vi "mfd_global.vi"() -> ()   [LabVIEW 2023]
panel:
  in  "MFD_GpsControl":T1
  out "MFD_Gps":picture
  in  "MFD_BatteryControl":T2
  in  "MFD_PowerControl":T3
  in  "MFD_RcControl":T4
  out "MFD_RadioBattery":picture
  in  "MFD_Stop":bool
  out "MFD_StatusText":picture
  in  "MFD_StatusTextControl":T5(array[cluster])
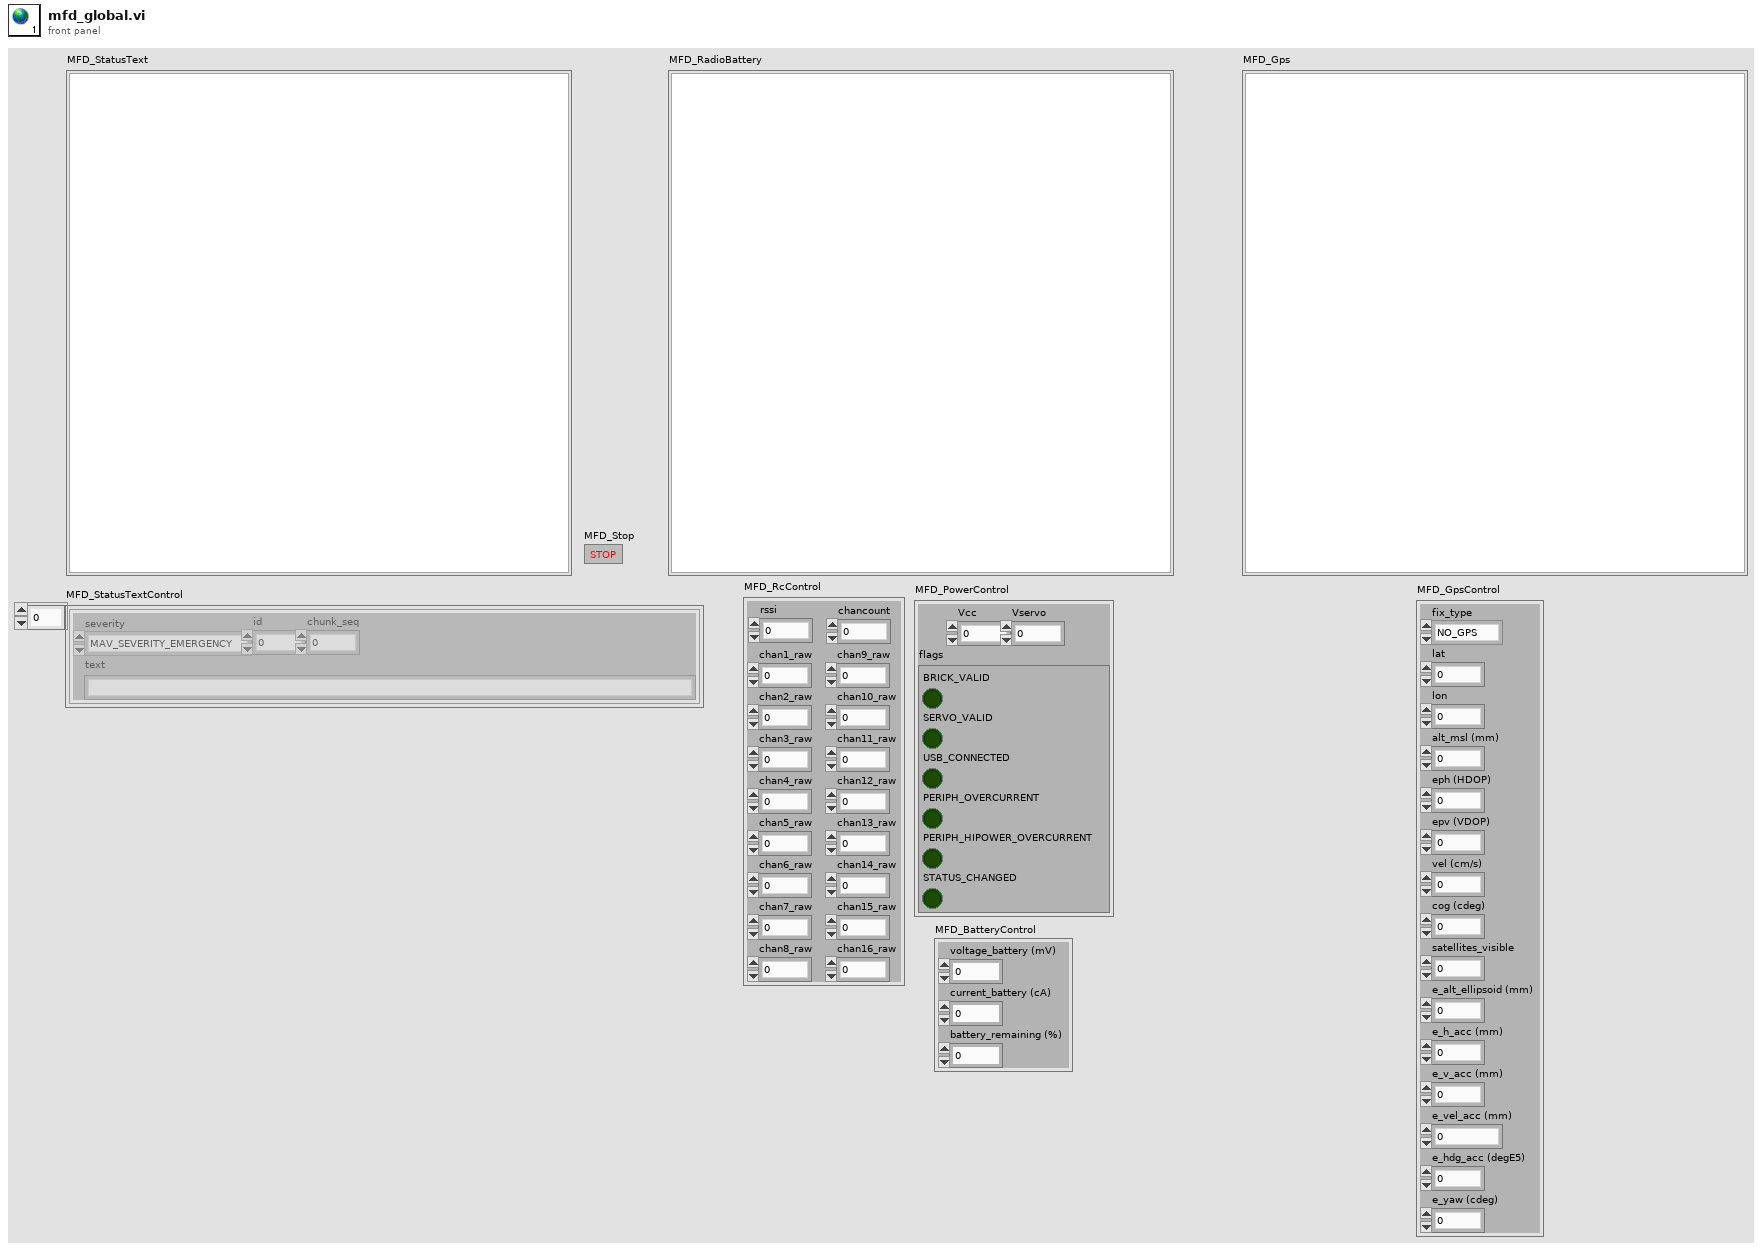
[diagram p1: front panel]
types:
  T1 = cluster{"lat":i32, "lon":i32, "alt_msl (mm)":i32, "eph (HDOP)":u16, "epv (VDOP)":u16, "vel (cm/s)":u16, "cog (cdeg)":u16, "satellites_visible":u8, "e_alt_ellipsoid (mm)":i32, "e_h_acc (mm)":u32, "e_v_acc (mm)":u32, "e_vel_acc (mm)":u32, "e_hdg_acc (degE5)":u32, "e_yaw (cdeg)":u16, "fix_type":enum16{"NO_GPS", "NO_FIX", "2D_FIX", "3D_FIX", "DGPS", "RTK_FLOAT", "RTK_FIXED", "STATIC", "PPP"}}
  T2 = cluster{"voltage_battery (mV)":u16, "current_battery (cA)":i16, "battery_remaining (%)":i8}
  T3 = cluster{"Vcc":u16, "Vservo":u16, "flags":cluster{"BRICK_VALID":bool, "SERVO_VALID":bool, "USB_CONNECTED":bool, "PERIPH_OVERCURRENT":bool, "PERIPH_HIPOWER_OVERCURRENT":bool, "STATUS_CHANGED":bool}}
  T4 = cluster{"chancount":u8, "chan1_raw":u16, "chan2_raw":u16, "chan3_raw":u16, "chan4_raw":u16, "chan5_raw":u16, "chan6_raw":u16, "chan7_raw":u16, "chan8_raw":u16, "chan9_raw":u16, "chan10_raw":u16, "chan11_raw":u16, "chan12_raw":u16, "chan13_raw":u16, "chan14_raw":u16, "chan15_raw":u16, "chan16_raw":u16, "rssi":u8}
  T5 = cluster{"severity":enum8{"MAV_SEVERITY_EMERGENCY", "MAV_SEVERITY_ALERT", "MAV_SEVERITY_CRITICAL", "MAV_SEVERITY_ERROR", "MAV_SEVERITY_WARNING", "MAV_SEVERITY_NOTICE", "MAV_SEVERITY_INFO", "MAV_SEVERITY_DEBUG"}, "id":u16, "chunk_seq":u8, "text":string}[]
diagram:
